vi "Query Resource Access Information - NPin MRsrc.vi"(7 "sites":i32[](array[numeric]), 8 "error in (no error)":errorcluster, 9 "instrument type id":string, 10 "pin or relay names":string[](array[string]), 11 "pin map id":string) -> (0 "error out":errorcluster, 2 "resource access information":T1[](array[typedef]))   [LabVIEW 2020, in "MeasurementLink Pin Map.lvlib"]
doc: "Queries the pin map service for resouce access information for the specified <b>pin or relay names</b>, <b>instrument type</b>, and <b>sites</b>. This information can be used to map pins to the associated hardware resources and connections used to make measurements on the pins."
uses:
  MeasurementLink Pin Map.lvlib
  MeasurementLink Pin Map Client/RPC Messages/ni_measurementlink_pinmap_v1_ResourceAccessInformation.ctl
  MeasurementLink Pin Map Client/RPC Messages/ni_measurementlink_pinmap_v1_ChannelMapping.ctl
  MeasurementLink gRPC Utilities/gRPC Client Pool/FGV Action.ctl
  MeasurementLink Pin Map Client/RPC Messages/ni_measurementlink_pinmap_v1_QueryResourceAccessInformationRequest.ctl
  MeasurementLink Measurement Server/Helpers/Error Strings Global Internal.vi
  MeasurementLink gRPC Utilities/gRPC Client Pool/gRPC Client Pool.lvclass
  MeasurementLink Pin Map Client/MeasurementLink Pin Map Client.lvlib
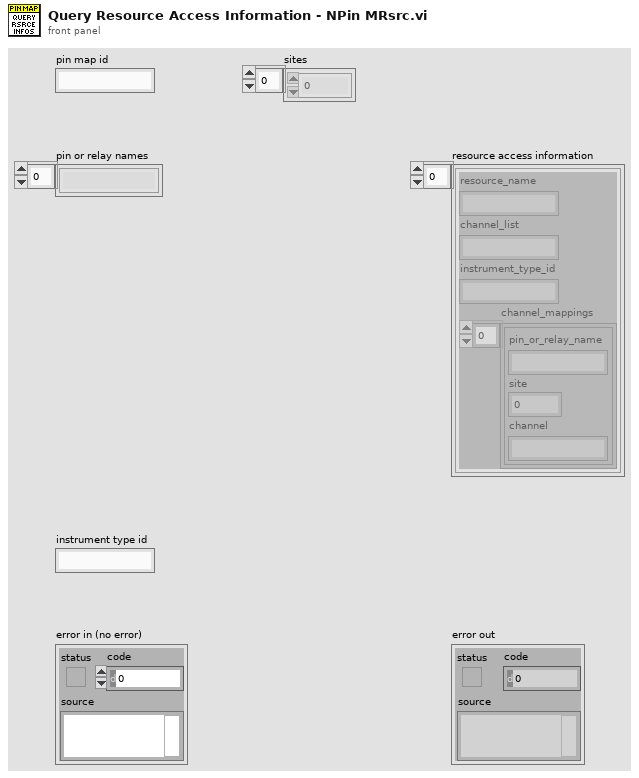
[diagram p1: front panel]
types:
  T1 = typedef "MeasurementLink Pin Map Client.lvlib/ni_measurementlink_pinmap_v1_ResourceAccessInformation.ctl" = cluster{"resource_name":string, "channel_list":string, "instrument_type_id":string, "channel_mappings":T2[]}
  T2 = typedef "MeasurementLink Pin Map Client.lvlib/ni_measurementlink_pinmap_v1_ChannelMapping.ctl" = cluster{"pin_or_relay_name":string, "site":i32, "channel":string}
  T3 = typedef "MeasurementLink Pin Map Client.lvlib/ni_measurementlink_pinmap_v1_QueryResourceAccessInformationRequest.ctl" = cluster{"pin_map_id":string, "sites":i32[], "pin_or_relay_names":string[], "instrument_type_id":string}
  T4 = typedef "MeasurementLink gRPC Utilities.lvlib/gRPC Client Pool.lvclass/FGV Action.ctl" = enum16{"Get Discovery Client", "Get Session Client", "Get Pinmap Client", "Destroy Clients"}
  T5 = typedef "grpc-lvsupport-release.lvlib/grpcId.ctl" = u64
  T6 = typedef "MeasurementLink Pin Map Client.lvlib/ni_measurementlink_pinmap_v1_QueryResourceAccessInformationResponse.ctl" = cluster{"resource_access_information":T1[]}
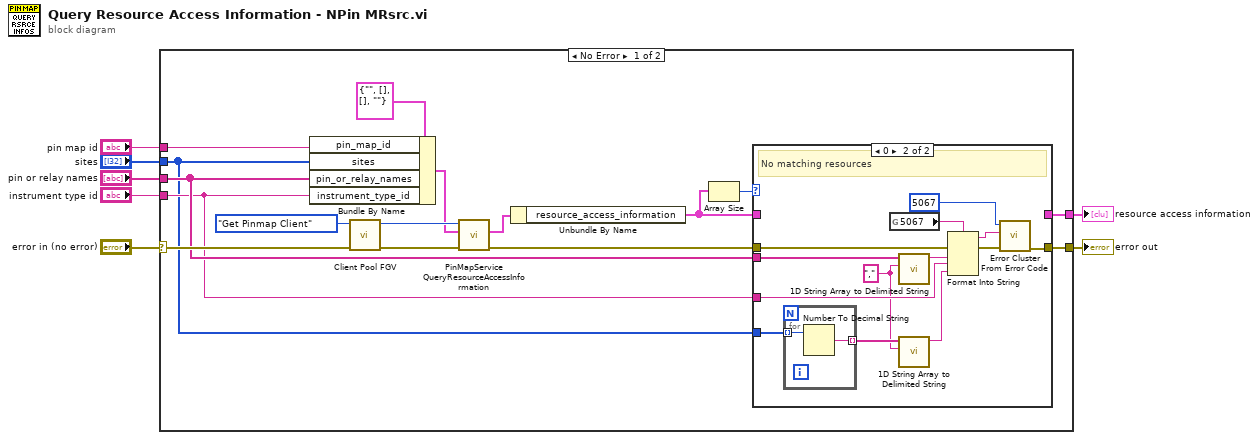
[diagram p0: block diagram]
diagram:
  n1 = case shown="No Error" "error in (no error)" {
    selector: "error in (no error)" -> [w17 w41]
    tunnel: "pin or relay names" -> [w10 _]
    tunnel: "instrument type id" -> [w9 _]
    tunnel: [w14 _] -> w5
    tunnel: [w11 w41] -> w4
    tunnel: "pin map id" -> [w16 _]
    tunnel: "sites" -> [w8 _]
    frame No Error {
      n2 = Bundle By Name(cluster=T3 {"pin_map_id"="", "sites"=[], "pin_or_relay_names"=[], "instrument_type_id"=""} ("Request Data"), "pin_map_id"=w16, "sites"=w8, "pin_or_relay_names"=w10, "instrument_type_id"=w9) -> (w19:T3)
      n3 = call "Client Pool FGV.vi"("error in (no error)"=w17, "Action"=FGV_Action."Get Pinmap Client") -> ("error out"=w22:errorcluster, "grpc client id"=w21:T5)  [unwired: 8 in]
      n4 = call "PinMapService QueryResourceAccessInformation.vi"("error in"=w22, "Request Data"=w19, "gRPC ID"=w21) -> ("error out"=w12:errorcluster, "Response Data"=w18:T6)  [unwired: 6 in, 1 out]
      n5 = Unbundle By Name(w18) -> ("resource_access_information"=w13:T1[])
      n6 = Array Size(array=w13) -> (size(s)=w15:i32)
      n7 = case shown="0" w15 {
        tunnel: [w25 _] -> w14
        tunnel: w13 -> [w25 _]
        tunnel: w12 -> [w24 w35]
        tunnel: [w24 w34] -> w11
        tunnel: w10 -> [_ w32]
        tunnel: w9 -> [_ w30]
        tunnel: w8 -> [_ w29]
        frame Default {
        }
        frame 0 {
          w27 = "," ("delimiter")
          # "No matching resources"
          n8 = for {
            tunnel: w29 -> [w40] mode=indexing
            tunnel: [w39] -> w28 mode=indexing
            n9 = Number To Decimal String(number=w40) -> (decimal integer string=w39:string)  [unwired: 1 in]
          }
          n10 = global read "Error Strings Global Internal.vi" "5067"() -> (w33:string)
          n11 = call <vilib>:"1D String Array to Delimited String.vi"("delimiter"=w27, "string array"=w32) -> ("delimited string"=w31:string)  [unwired: 9 in]
          n12 = call <vilib>:"1D String Array to Delimited String.vi"("delimiter"=w27, "string array"=w28) -> ("delimited string"=w26:string)  [unwired: 9 in]
          n13 = Format Into String(format string=w33, error in=w35, w31, w30, w26) -> (resulting string=w36:string, error out=w37:errorcluster)  [unwired: 1 in]
          n14 = call <vilib>:"Error Cluster From Error Code.vi"("error in (no error)"=w37, "error message (\"\")"=w36, "error code (0)"=5067) -> ("error out"=w34:errorcluster)  [unwired: 6 in]
        }
      }
    }
    frame Error {
    }
  }
  "error out" <- w4
  "resource access information" <- w5
